vi "Configure Modulation(Frequency).vi"(0 "VISA resource name":refnum<visa-resource-name>, 1 "Enable Frequency Modulation (F: Disable)":bool, 2 "Frequency Deviation (1000 Hz)":dbl=1000.0, 5 "Channel (1: Channel 1)":i32(ring)=1 items=["Channel 1"=1, "Channel 2"=2], 7 "FM Source (0: Internal)":i32(ring) items=["Internal", "External"], 9 "Modulation Waveform (0: Sinusoid)":i32(ring) items=["Sinusoid", "Square", "Triangle", "Ramp", "Nramp", "Noise", "User"], 11 "error in (no error)":errorcluster, 12 "Modulation Frequency (100 Hz)":dbl=100.0) -> (4 "VISA resource name out":refnum<visa-resource-name>, 15 "error out":errorcluster)   [LabVIEW 2012, in "RIGOL DG4000 Series.lvlib"]
doc: "Configures frequency modulation."
uses:
  <instrlib>/RIGOL DG4000 Series/RIGOL DG4000 Series.lvlib
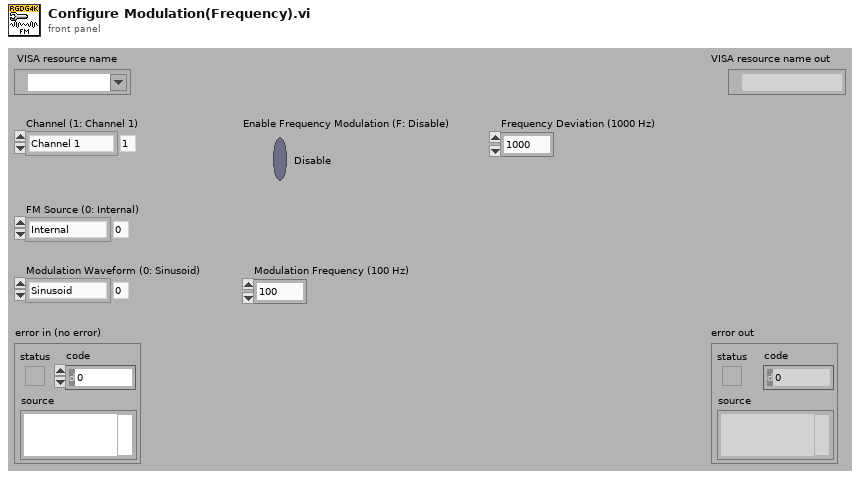
[diagram p1: front panel]
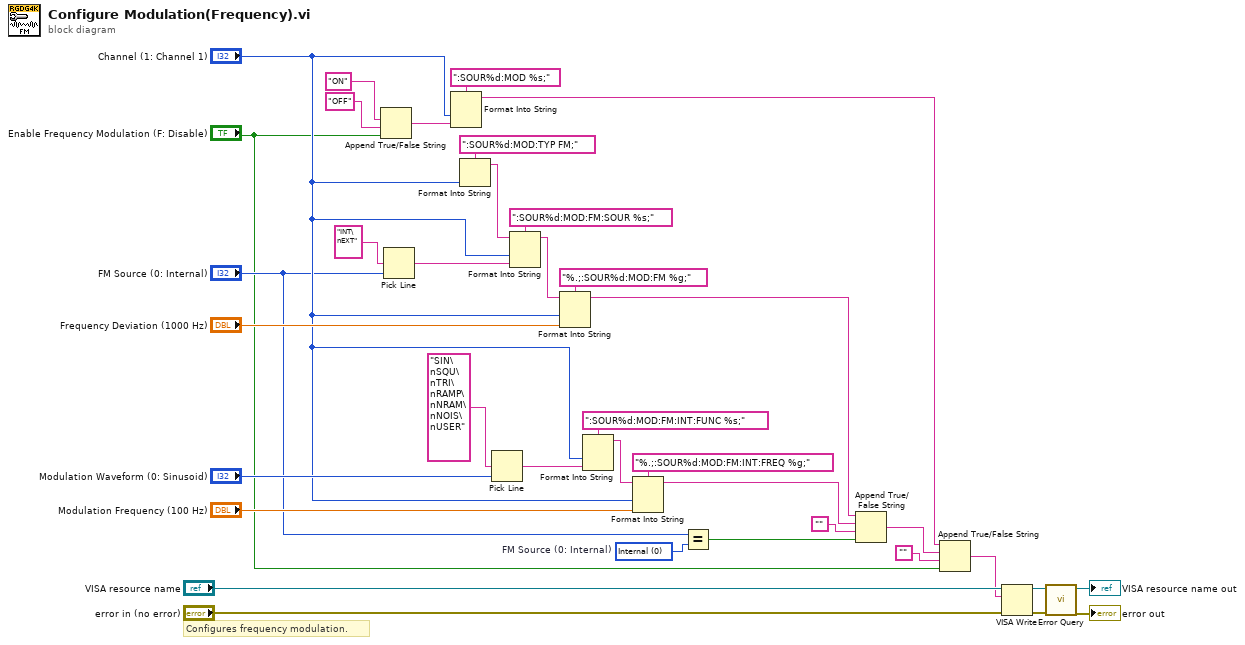
[diagram p0: block diagram]
diagram:
  w7 = 0 items=["Internal", "External"]  # FM Source (0: Internal)
  # "Configures frequency modulation."
  n1 = Append True/False String(1:"Enable Frequency Modulation (F: Disable)", 2:"OFF", 3:"ON") -> (0:w34:string)  [unwired: 1 out]
  n2 = Pick Line(multi-line string="INT\nEXT", line index="FM Source (0: Internal)") -> (output string=w29:string)  [unwired: 1 out]
  n3 = Format Into String(format string=":SOUR%d:MOD %s;", "Channel (1: Channel 1)", w34) -> (resulting string=w4:string)  [unwired: 2 in, 1 out]
  n4 = Format Into String(format string=":SOUR%d:MOD:TYP FM;", "Channel (1: Channel 1)") -> (resulting string=w31:string)  [unwired: 2 in, 1 out]
  n5 = Pick Line(multi-line string="SIN\nSQU\nTRI\nRAMP\nNRAM\nNOIS\nUSER", line index="Modulation Waveform (0: Sinusoid)") -> (output string=w23:string)  [unwired: 1 out]
  n6 = Format Into String(format string=":SOUR%d:MOD:FM:SOUR %s;", initial string=w31, "Channel (1: Channel 1)", w29) -> (resulting string=w13:string)  [unwired: 1 in, 1 out]
  n7 = Format Into String(format string="%.;:SOUR%d:MOD:FM %g;", initial string=w13, "Channel (1: Channel 1)", "Frequency Deviation (1000 Hz)") -> (resulting string=w12:string)  [unwired: 1 in, 1 out]
  n8 = Format Into String(format string=":SOUR%d:MOD:FM:INT:FUNC %s;", "Channel (1: Channel 1)", w23) -> (resulting string=w22:string)  [unwired: 2 in, 1 out]
  n9 = Format Into String(format string="%.;:SOUR%d:MOD:FM:INT:FREQ %g;", initial string=w22, "Channel (1: Channel 1)", "Modulation Frequency (100 Hz)") -> (resulting string=w11:string)  [unwired: 1 in, 1 out]
  n10 = Equal?(x="FM Source (0: Internal)", y=w7) -> (x = y?=w9:bool)
  n11 = Append True/False String(1:w9, 2:"", 3:w11, 4:w12) -> (0:w3:string)
  n12 = Append True/False String(1:"Enable Frequency Modulation (F: Disable)", 2:"", 3:w3, 4:w4) -> (0:w1:string)
  n13 = VISA Write(VISA resource name="VISA resource name", write buffer=w1, error in (no error)="error in (no error)") -> (VISA resource name out=w17:refnum<visa-resource-name>, error out=w16:errorcluster)  [unwired: 1 out]
  n14 = call <instrlib>:"Error Query.vi"("error in (no error)"=w16, "VISA resource name"=w17) -> ("error out"=→"error out":errorcluster, "VISA resource name out"=→"VISA resource name out":refnum<visa-resource-name>)  [unwired: 8 out]
